vi "Set Exposure Time.vi"(8 "error in (no error)":errorcluster, 10 "Exposure Time (s)":dbl, 11 "Simulated in":refnum<class "Simulated.lvclass">) -> (0 "error out":errorcluster, 2 "Exposure Time (s) out":dbl, 3 "Simulated out":refnum<class "Simulated.lvclass">)   [LabVIEW 2019, in "Simulated.lvclass"]
uses:
  Simulated.lvclass
  Simulated.lvclass/Simulated.ctl
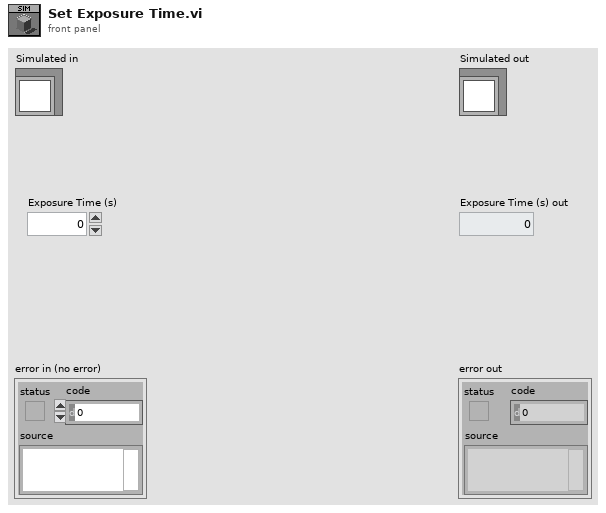
[diagram p1: front panel]
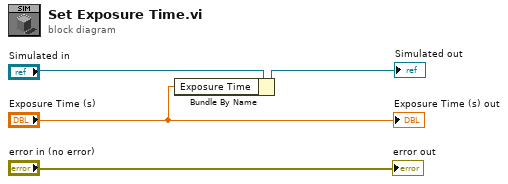
[diagram p0: block diagram]
diagram:
  n1 = Bundle By Name(cluster="Simulated in", "Exposure Time"="Exposure Time (s)") -> (→"Simulated out":refnum<class "Simulated.lvclass">)
  "error out" <- "error in (no error)"
  "Exposure Time (s) out" <- "Exposure Time (s)"
